vi "trapezoidal_control.vi"() -> ()   [LabVIEW 2020]
uses:
  <vilib>/Analysis/1siggen.llb/Ramp Pattern by Samples.vi
  <vilib>/Analysis/NI_AALBase.lvlib
panel:
  in  "Offset 2":dbl(slide) min=-8.0 max=8.0 step=1.0 scale=-8.0..8.0
  in  "Amplitude 2":dbl(knob) min=0.0 max=10.0 step=1.0 scale=0.0..10.0
  out "Waveform Pattern":dbl[](graph)
  in  "Stop":bool
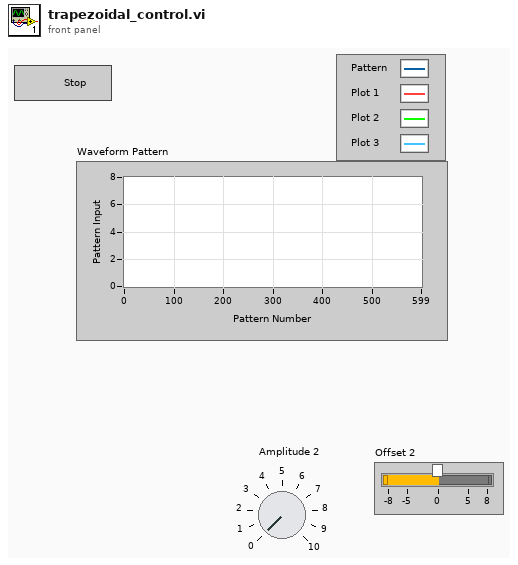
[diagram p1: front panel]
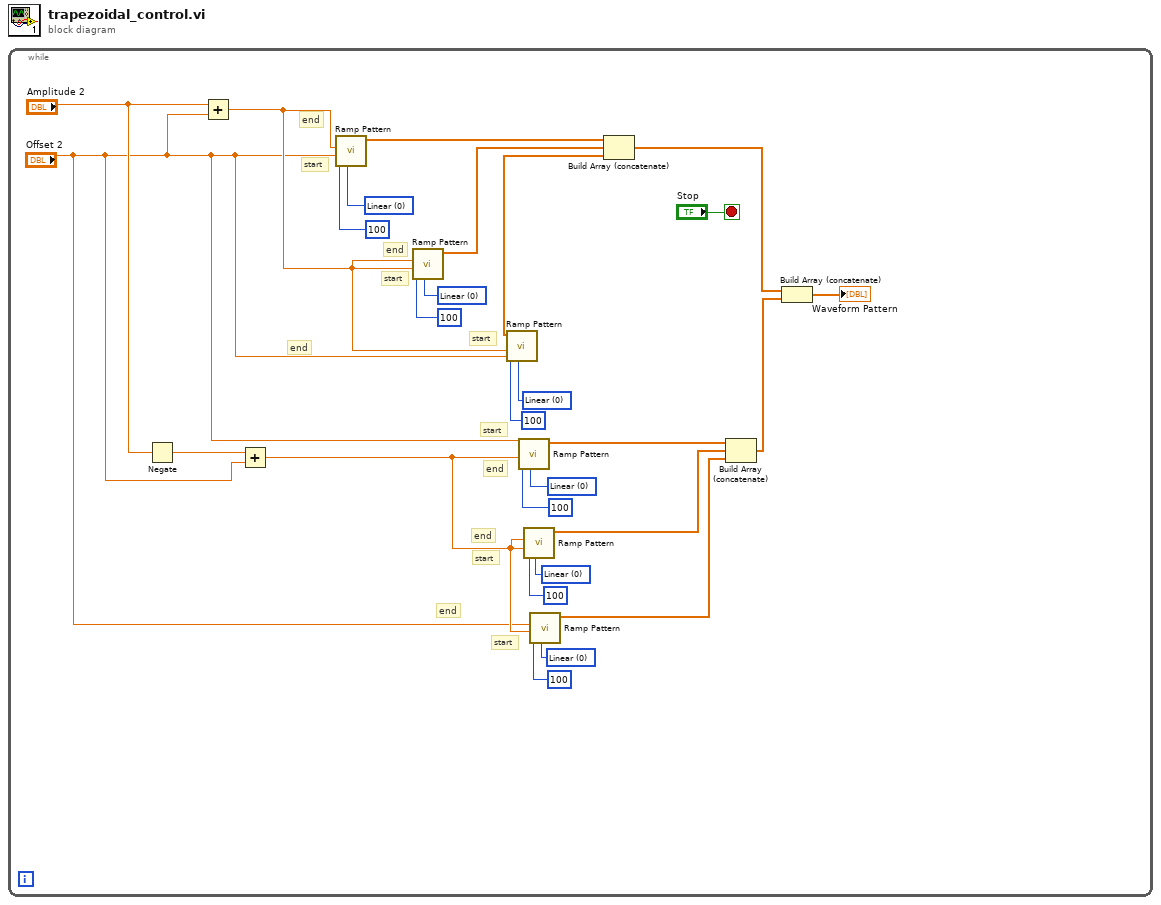
[diagram p0: block diagram]
diagram:
  n1 = while {
    stop <- "Stop" stop-if-true
    w6 = u16 0 items=["Linear", "Logarithmic"] ("type")
    w7 = u16 0 items=["Linear", "Logarithmic"] ("type")
    w13 = u16 0 items=["Linear", "Logarithmic"] ("type")
    w11 = u16 0 items=["Linear", "Logarithmic"] ("type")
    w24 = u16 0 items=["Linear", "Logarithmic"] ("type")
    w26 = u16 0 items=["Linear", "Logarithmic"] ("type")
    # "start"
    # "end"
    # "end"
    # "start"
    # "start"
    # "end"
    # "end"
    # "start"
    # "start"
    # "end"
    # "end"
    # "start"
    n2 = Negate(x="Amplitude 2") -> (-x=w3:dbl)
    n3 = Add(x="Amplitude 2", y="Offset 2") -> (x+y=w5:dbl)
    n4 = Add(x=w3, y="Offset 2") -> (x+y=w2:dbl)
    n5 = call-poly <vilib>:"Ramp Pattern.vi"("type"=w26, "start"="Offset 2", "end"=w5, "samples"=100) -> ("Ramp Pattern"=w21:dbl[])  [unwired: 6 in, 1 out]
    n6 = call-poly <vilib>:"Ramp Pattern.vi"("type"=w24, "start"=w5, "end"=w5, "samples"=100) -> ("Ramp Pattern"=w22:dbl[])  [unwired: 6 in, 1 out]
    n7 = call-poly <vilib>:"Ramp Pattern.vi"("type"=w7, "start"=w5, "end"="Offset 2", "samples"=100) -> ("Ramp Pattern"=w19:dbl[])  [unwired: 6 in, 1 out]
    n8 = call-poly <vilib>:"Ramp Pattern.vi"("type"=w11, "start"="Offset 2", "end"=w2, "samples"=100) -> ("Ramp Pattern"=w16:dbl[])  [unwired: 6 in, 1 out]
    n9 = call-poly <vilib>:"Ramp Pattern.vi"("type"=w13, "start"=w2, "end"=w2, "samples"=100) -> ("Ramp Pattern"=w15:dbl[])  [unwired: 6 in, 1 out]
    n10 = call-poly <vilib>:"Ramp Pattern.vi"("type"=w6, "start"=w2, "end"="Offset 2", "samples"=100) -> ("Ramp Pattern"=w18:dbl[])  [unwired: 6 in, 1 out]
    n11 = Build Array (concatenate)(w21, w22, w19) -> (w10:dbl[])
    n12 = Build Array (concatenate)(w16, w15, w18) -> (w9:dbl[])
    n13 = Build Array (concatenate)(w10, w9) -> (→"Waveform Pattern":dbl[])
  }
